vi "Initialise.vi"(8 "error in (no error)":errorcluster, 10 "Message in":refnum<class "InitialiseMessage.lvclass">, 11 "Cascade in":refnum<class "Cascade.lvclass">) -> (0 "error out":errorcluster, 3 "Cascade out":refnum<class "Cascade.lvclass">)   [LabVIEW 2012, in "Cascade.lvclass"]
doc: "This method is called when an initialise message is received. It mainly initialises the RabbitMQ connectivity. \n\nOverride this method when your component needs special initialisation (e.g. of software or hardware resources). In that case, don't forget to call the parent for proper implementation. If your component owns subcomponents, they count as resources, so you have to initialise them by calling their own initialise functions"
uses:
  Cascade.lvclass
  <vilib>/Distrio/Murmex/InitialiseMessage/InitialiseMessage.lvclass
  <vilib>/Distrio/Murmex/Murmex/Murmex.lvclass
  data type.ctl
  Cascade.lvclass/Cascade.ctl
panel:
  # "This method is called when the INTIALISE\ntrigger is sent. \n\nOverride this method when your component needs to\nrespond to this trigger. \n\nCall parent for proper implementation"
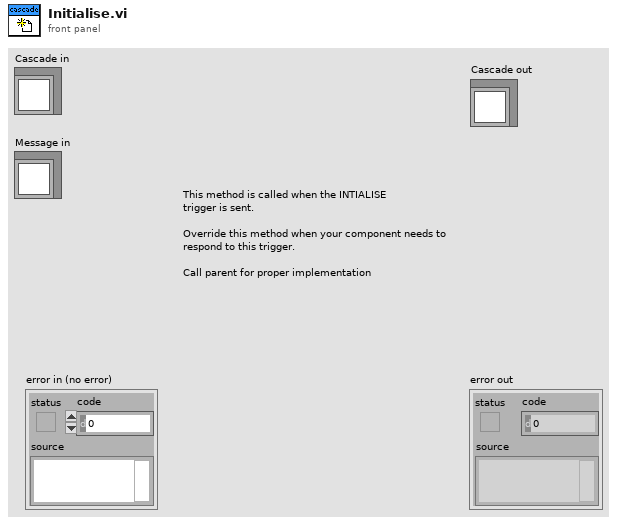
[diagram p1: front panel]
types:
  T1 = typedef "Cascade.lvclass/data type.ctl" = u32
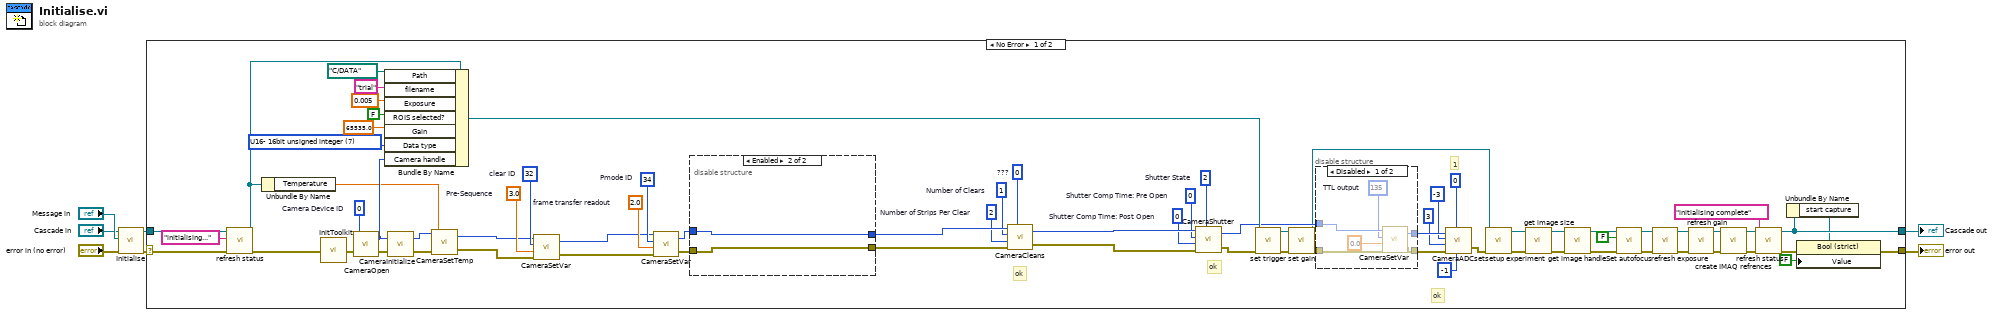
[diagram p0: block diagram]
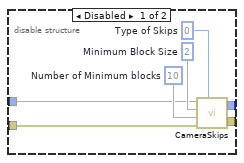
[diagram p2: hidden frame]
diagram:
  n1 = call-parent "Initialise.vi"("error in (no error)"="error in (no error)", "Message in"="Message in", "Murmex in"="Cascade in") -> ("error out"=w4:errorcluster, "Murmex out"=w3:refnum<class "Cascade.lvclass">)  [unwired: 7 in]
  n2 = case shown="No Error" w4 {
    selector: w4 -> [w35 w99]
    tunnel: w3 -> [w33 w98]
    tunnel: [w25 w99] -> w2
    tunnel: [w28 w98] -> w1
    frame No Error {
      w60 = 2.0  # frame transfer readout
      w59 = u32 34  # Pmode ID
      w58 = 3.0  # Pre-Sequence
      w57 = u32 32  # clear ID
      w66 = T1 7 items=["8bit signed integer"=1, "I16- 16bit signed integer"=2, "I32- 32bit signed integer"=3, "SGL- 32 bit floating point"=4, "DBL- 64 bit floating point"=5, "U8- 8bit unsigned"=6, "U16- 16bit unsigned integer"=7, "U32- 32 bit unsigned integer"=8] ("runtime.Data type")
      w69 = u32 0  # Shutter Comp Time: Post Open
      w70 = u32 0  # Shutter Comp Time: Pre Open
      w71 = u32 2  # Shutter State
      w72 = u32 2  # Number of Strips Per Clear
      w73 = u32 1  # Number of Clears
      w74 = u32 0  # ???
      w79 = u32 0  # Camera Device ID
      # "ok"
      # "ok"
      # "ok"
      # "1"
      n3 = call-dynamic "refresh status.vi"("error in (no error)"=w35, "String In"="initialising...", "Cascade in"=w33) -> ("error out"=w34:errorcluster, "Cascade out"=w32:refnum<class "Cascade.lvclass">)  [unwired: 7 in]
      n4 = Unbundle By Name(w32) -> ("Temperature"=w61:dbl)
      n5 = call <userlib>:"InitToolkit.vi"("error in"=w34) -> ("error out"=w80:errorcluster)
      n6 = call <userlib>:"CameraOpen.vi"("error in"=w80, "Camera Device ID"=w79) -> ("error out"=w65:errorcluster, "Camera Handle"=w64:u32)
      n7 = Bundle By Name(cluster=w32, "Path"=path "C:/DATA" ("settings.Path"), "filename"="trial" ("settings.filename"), "Exposure"=dbl[unit] 0.005 ("settings.Exposure"), "ROIS selected?"=FALSE ("runtime.ROIS selected?"), "Gain"=65535.0 ("settings.Gain"), "Data type"=w66, "Camera handle"=w64) -> (w67:refnum<class "Cascade.lvclass">)
      n8 = call <userlib>:"CameraInitialize.vi"("error in"=w65, "Camera Handle"=w64) -> ("error out"=w63:errorcluster, "Camera Handle"=w62:u32)
      n9 = call <userlib>:"CameraSetTemp.vi"("error in (no error)"=w63, "Temperature"=w61, "Camera Handle"=w62) -> ("error out"=w54:errorcluster, "Camera Handle"=w53:u32)
      n10 = call <userlib>:"CameraSetVar.vi"("error in"=w54, "Value"=w58, "Parameter ID"=w57, "Camera Handle"=w53) -> ("error out"=w55:errorcluster, "CameraHandle"=w56:u32)
      n11 = call <userlib>:"CameraSetVar.vi"("error in"=w55, "Value"=w60, "Parameter ID"=w59, "Camera Handle"=w56) -> ("error out"=w52:errorcluster, "CameraHandle"=w51:u32)
      n12 = disable-structure shown="Enabled" {
        disable-tunnel: [w87 w89] -> w78
        disable-tunnel: [w86 w88] -> w77
        disable-tunnel: w52 -> [w82 w88]
        disable-tunnel: w51 -> [w81 w89]
        frame Disabled {
          w83 = u32 0  # Type of Skips
          w84 = u32 10  # Number of Minimum blocks
          w85 = u32 2  # Minimum Block Size
          n13 = call <userlib>:"CameraSkips.vi"("Camera Handle"=w81, "Minimum Block Size"=w85, "Number of Minimum blocks"=w84, "error in"=w82, "Type of Skips"=w83) -> ("Camera Handle"=w87:u32, "error out"=w86:errorcluster)
        }
        frame Enabled {
        }
      }
      n14 = call <userlib>:"CameraCleans.vi"("Camera Handle"=w78, "Number of Clears"=w73, "Number of Strips Per Clear"=w72, "error in"=w77, "Continuous Clears"=w74) -> ("Camera Handle"=w75:u32, "error out"=w76:errorcluster)
      n15 = call <userlib>:"CameraShutter.vi"("Camera Handle"=w75, "Shutter Comp Time: Pre Open"=w70, "Shutter Comp Time: Post Open"=w69, "error in"=w76, "Shutter State"=w71) -> ("Camera Handle"=w50:u32, "error out"=w68:errorcluster)
      n16 = call-dynamic "set trigger.vi"("error in (no error)"=w68, "Cascade in"=w67) -> ("error out"=w17:errorcluster, "Cascade out"=w15:refnum<class "Cascade.lvclass">)  [unwired: 8 in]
      n17 = call-dynamic "set gain.vi"("error in (no error)"=w17, "Cascade in"=w15) -> ("error out"=w16:errorcluster, "Cascade out"=w14:refnum<class "Cascade.lvclass">)  [unwired: 8 in]
      n18 = disable-structure shown="Disabled" {
        disable-tunnel: w50 -> [w95 w97]
        disable-tunnel: [w92 w96] -> w49
        disable-tunnel: [w91 w97] -> w48
        disable-tunnel: w16 -> [w90 w96]
        frame Disabled {
          w94 = u32 135  # TTL output
          n19 = call <userlib>:"CameraSetVar.vi"("error in"=w90, "Value"=0.0, "Parameter ID"=w94, "Camera Handle"=w95) -> ("error out"=w92:errorcluster, "CameraHandle"=w91:u32)
        }
        frame Enabled {
        }
      }
      n20 = call <userlib>:"CameraADCset.vi"("ADC offset"=-1, "Read Out port"=0, "error in (no error)"=w49, "ADC Gain"=3, "ADC Speed"=-3, "Camera Handle"=w48) -> ("error out"=w39:errorcluster)  [unwired: 1 out]
      n21 = call-dynamic "setup experiment.vi"("error in (no error)"=w39, "Cascade in"=w14) -> ("error out"=w44:errorcluster, "Cascade out"=w42:refnum<class "Cascade.lvclass">)  [unwired: 8 in]
      n22 = call-dynamic "get image size.vi"("error in (no error)"=w44, "Cascade in"=w42) -> ("error out"=w43:errorcluster, "Cascade out"=w41:refnum<class "Cascade.lvclass">)  [unwired: 8 in]
      n23 = call-dynamic "get image handle.vi"("error in (no error)"=w43, "Cascade in"=w41) -> ("error out"=w21:errorcluster, "Cascade out"=w12:refnum<class "Cascade.lvclass">)  [unwired: 8 in]
      n24 = call-dynamic "Set autofocus.vi"("error in (no error)"=w21, "autofocusing?"=FALSE, "Cascade in"=w12) -> ("error out"=w13:errorcluster, "Cascade out"=w11:refnum<class "Cascade.lvclass">)  [unwired: 7 in]
      n25 = call-dynamic "refresh exposure.vi"("error in (no error)"=w13, "Cascade in"=w11) -> ("error out"=w20:errorcluster, "Cascade out"=w22:refnum<class "Cascade.lvclass">)  [unwired: 8 in]
      n26 = call-dynamic "refresh gain.vi"("error in (no error)"=w20, "Cascade in"=w22) -> ("error out"=w37:errorcluster, "Cascade out"=w36:refnum<class "Cascade.lvclass">)  [unwired: 8 in]
      n27 = call-dynamic "create IMAQ refrences.vi"("error in (no error)"=w37, "Cascade in"=w36) -> ("error out"=w18:errorcluster, "Cascade out"=w19:refnum<class "Cascade.lvclass">)  [unwired: 8 in]
      n28 = call-dynamic "refresh status.vi"("error in (no error)"=w18, "String In"="initialising complete", "Cascade in"=w19) -> ("error out"=w26:errorcluster, "Cascade out"=w28:refnum<class "Cascade.lvclass">)  [unwired: 7 in]
      n29 = Unbundle By Name(w28) -> ("start capture"=w27:refnum<vi>)
      n30 = property class="Bool (strict)"(reference=w27, error in=w26, "Value"=FALSE) -> (error out=w25:errorcluster)  [unwired: 1 out]
    }
    frame Error {
    }
  }
  "error out" <- w2
  "Cascade out" <- w1
